vi "GraphMonitor.vi"(8 "error in (no error)":errorcluster, 11 "Connection ID":T2) -> (0 "error out":errorcluster, 3 "Connection ID Out":T2)   [LabVIEW 2017, in "GL860_Driver.lvlib"]
uses:
  GL860_Driver.lvlib
  Driver/ConnectionID.ctl
  D:/src/LabVIEW/GL860/JP/LabView VI/64bitdll/GLSampleProgram.dll
  64bitdll/GLSampleProgram.dll
  Sub/Amp_Param.ctl
panel:
  out "M/C":i32[](array[numeric])
  in  "HEAD":T1 {"FirstPos" format="%<%x %.3X>T"; "Stop" format="%<%x %.3X>T"; "Trig" format="%<%x %.3X>T"; "Start" format="%<%x %.3X>T"}
  out "LogiPul":i32
  out "MaxCH":i32
  out "Unit":bool[](array[boolean])
  out "Bin":i32[](array[numeric])
  out "Reference":refnum<k24>
  out "Pos":i32[](array[numeric])
  out "Idx":i32[](array[numeric])
  out "CH_Size":cluster{"Analog":i32, "Logic":i16, "Pulse":i16}
  in  "閉じる":bool
  in  "一時停止":bool
  out "カーソル値":string
  in  "Ch Select":u16(ring)
  out "Graph":dbl[][](graph)
  # "ALL"
  # "GBD"
  # "CSV"
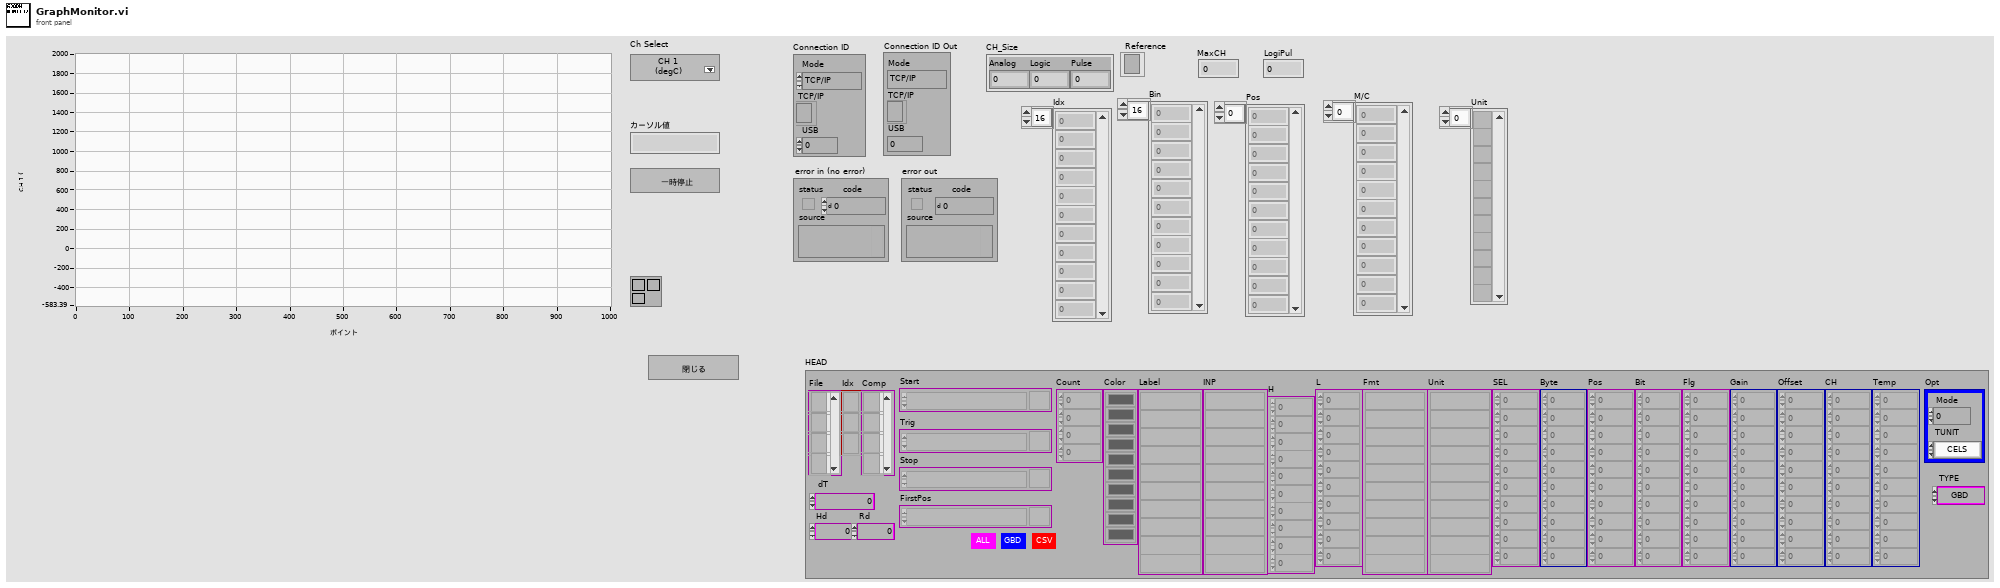
[diagram p1: front panel]
types:
  T1 = typedef "Amp_Param.ctl" = cluster{"File":refnum<file>[], "Idx":refnum<file>[], "dT":dbl, "Hd":i32, "Rd":i32, "Start":timestamp[], "Trig":timestamp[], "Stop":timestamp[], "FirstPos":timestamp[], "Count":i64[], "Color":u32[], "Label":string[], "INP":string[], "H":dbl[], "L":dbl[], "Fmt":string[], "Unit":string[], "SEL":i32[], "Byte":i32[], "Pos":i32[], "Bit":i32[], "Flg":i32[], "Gain":dbl[], "Offset":dbl[], "CH":i32[], "Opt":cluster{"Mode":i32, "TUNIT":enum16{"CELS", "FAHR"}}, "TYPE":enum16{"GBD", "CSV"}, "Comp":refnum<file>[], "Temp":i32[]}
  T2 = typedef "ConnectionID.ctl" = cluster{"Mode":enum16{"TCP/IP", "USB"}, "TCP/IP":refnum<k5>, "USB":i32}
  T3 = cluster{"Meas.Hi":string, "Meas.Lo":string, "Meas.Unit":string, "EU.Hi":string, "EU.Lo":string, "EU.Unit":string}
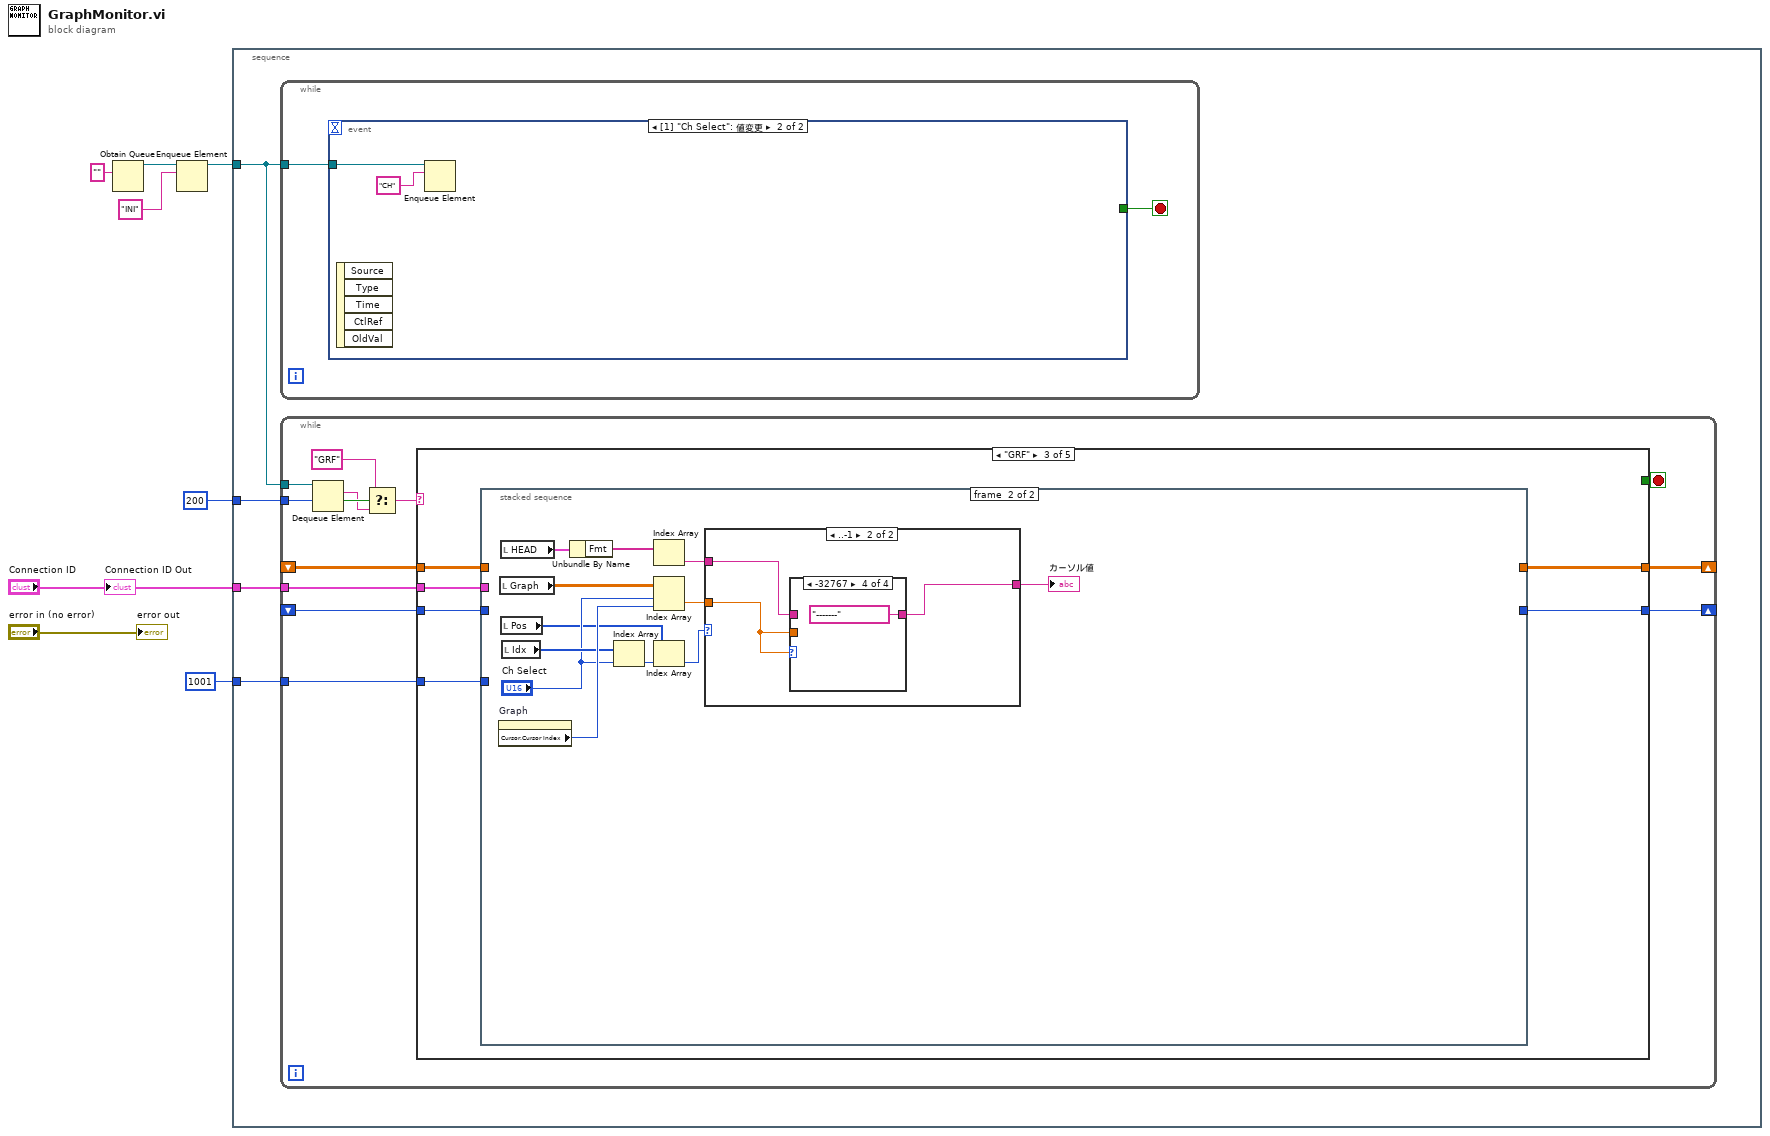
[diagram p0: block diagram]
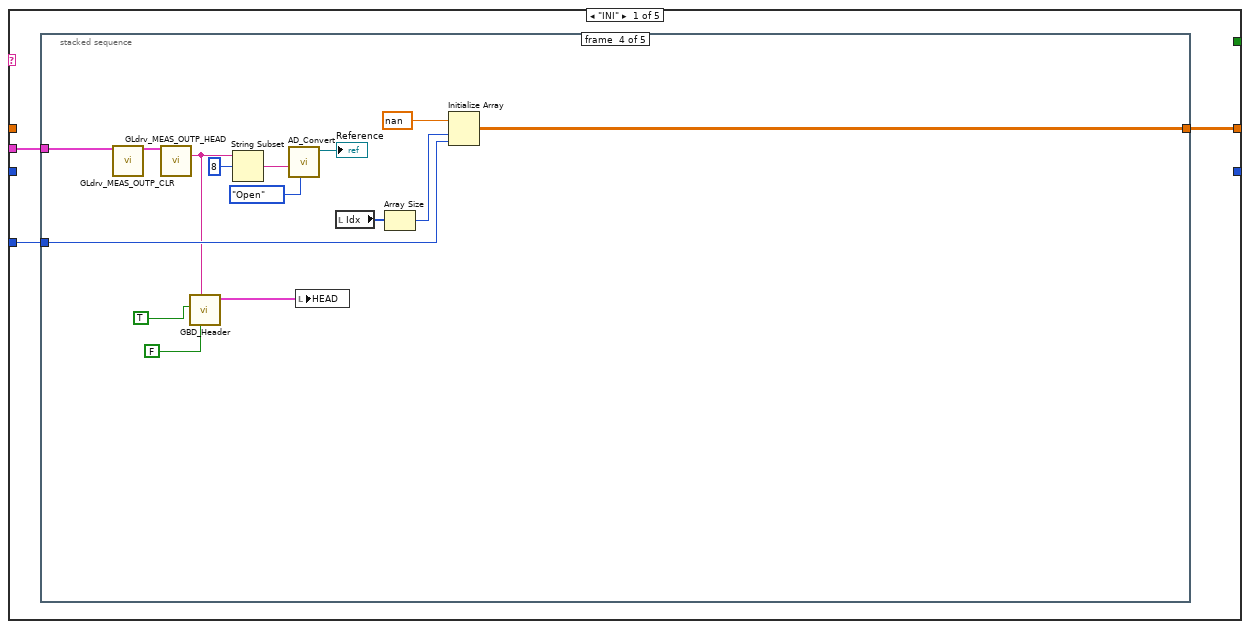
[diagram p2: hidden frame]
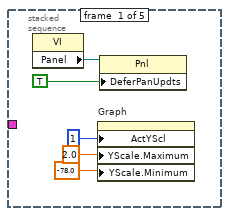
[diagram p3: hidden frame]
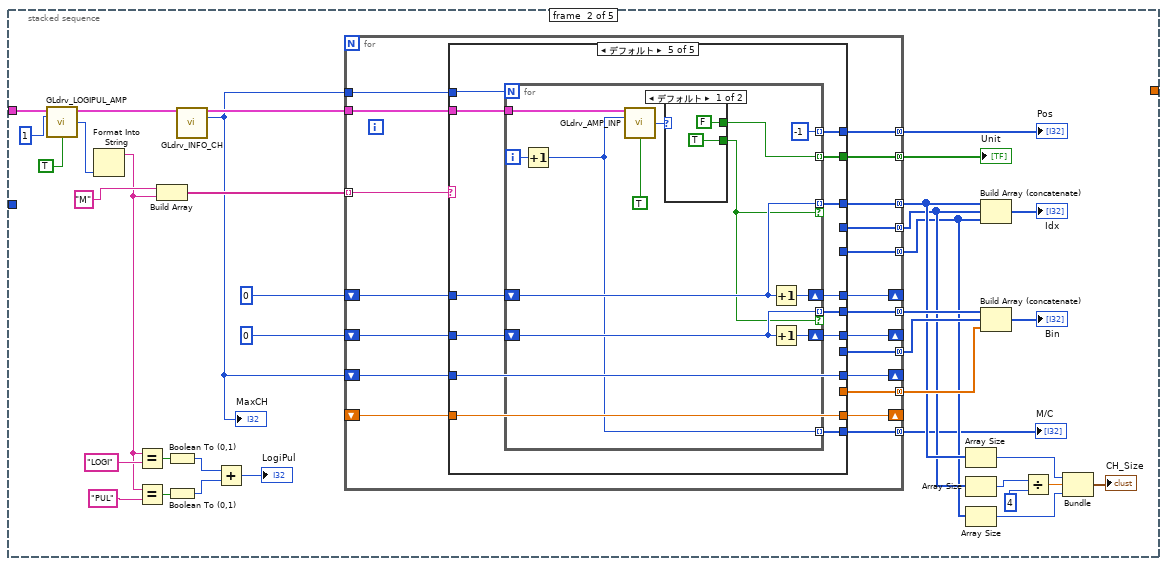
[diagram p4: hidden frame]
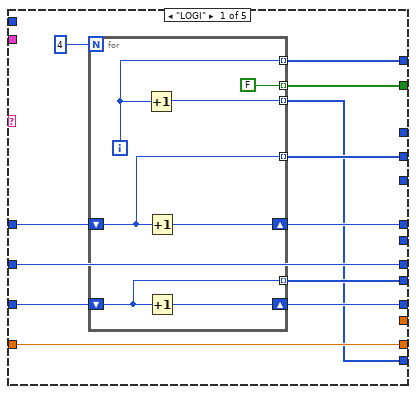
[diagram p5: hidden frame]
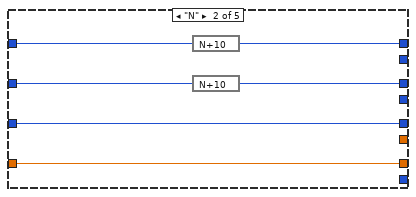
[diagram p6: hidden frame]
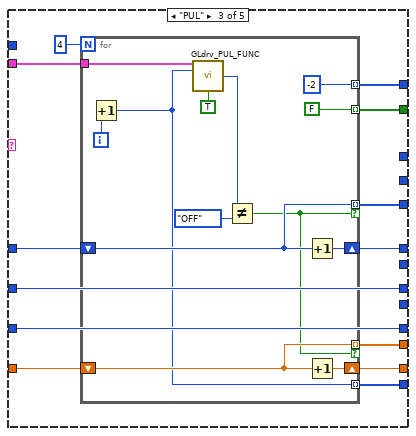
[diagram p7: hidden frame]
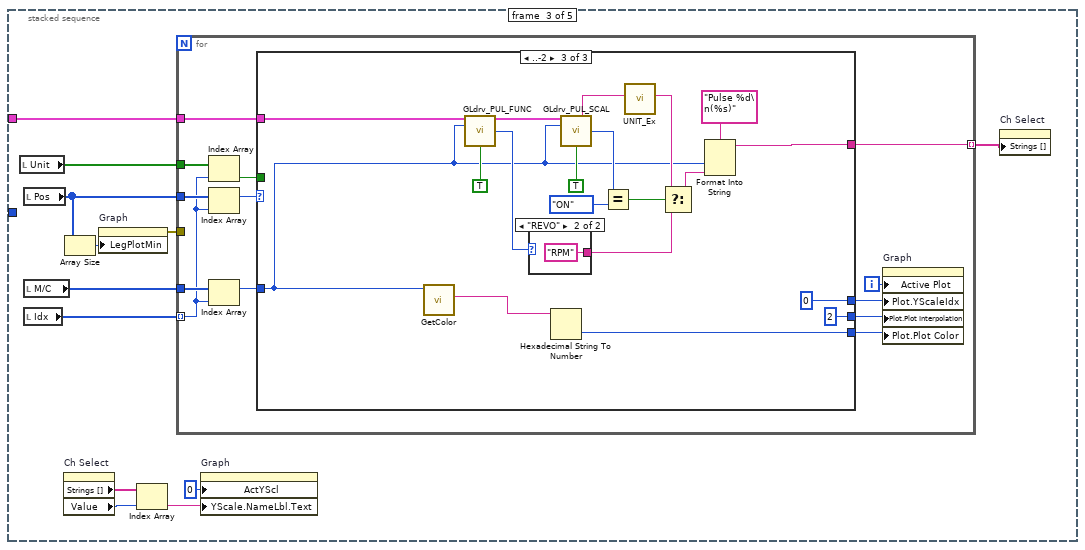
[diagram p10: hidden frame]
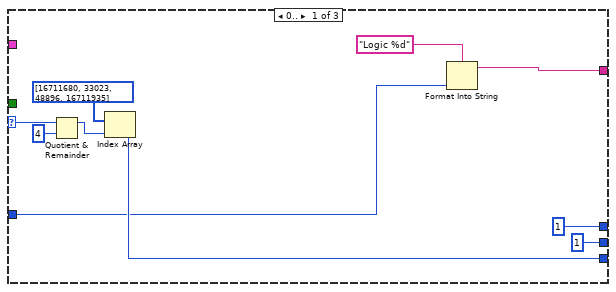
[diagram p11: hidden frame]
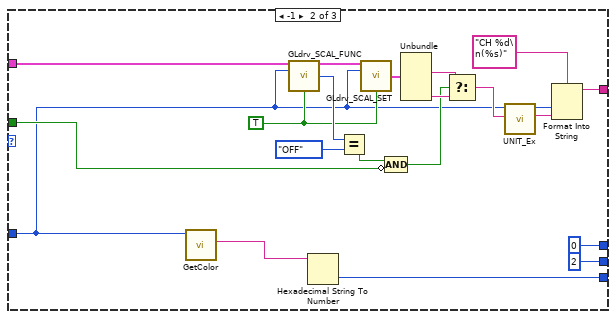
[diagram p12: hidden frame]
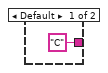
[diagram p13: hidden frame]
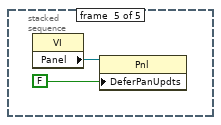
[diagram p14: hidden frame]
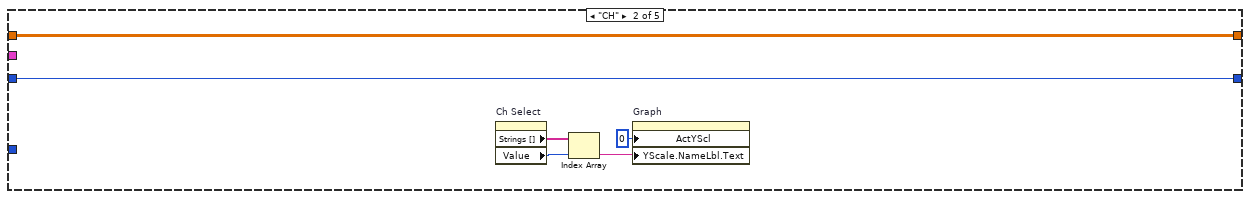
[diagram p15: hidden frame]
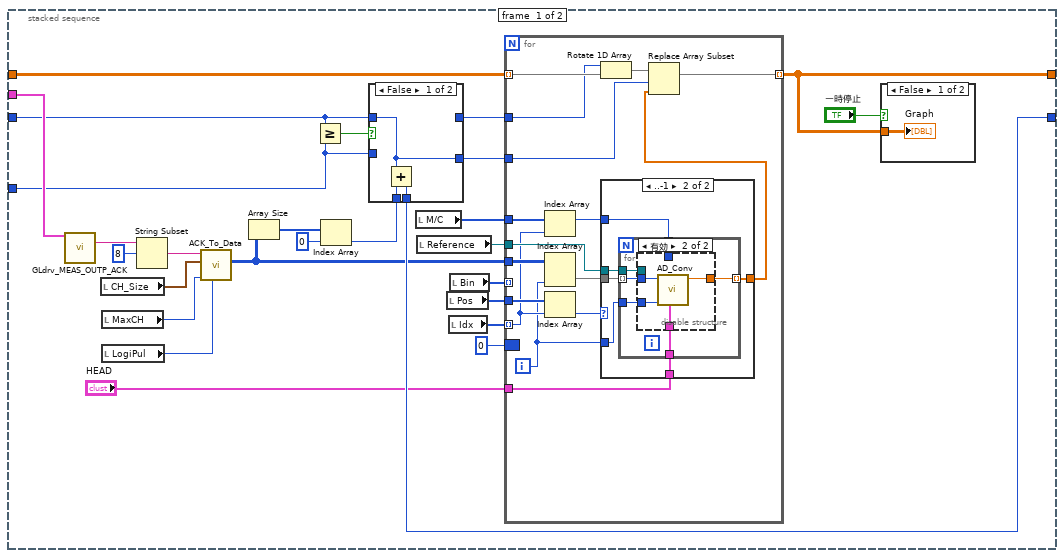
[diagram p16: hidden frame]
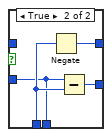
[diagram p18: hidden frame]
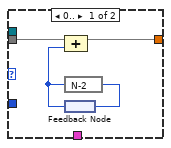
[diagram p19: hidden frame]
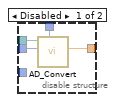
[diagram p20: hidden frame]
diagram:
  n1 = Obtain Queue(element data type="") -> (queue out=w4:refnum<queue>)  [unwired: 4 in, 2 out]
  n2 = Enqueue Element(queue=w4, element="INI") -> (queue out=w3:refnum<queue>)  [unwired: 2 in, 2 out]
  n3 = stacked-sequence {
    tunnel: "Connection ID" -> [w12]
    tunnel: w3 -> [w11]
    tunnel: 200 -> [w10]
    tunnel: 1001 ("dimension size") -> [w9]
    frame #0 {
      n4 = while {
        tunnel: w11 -> [w382]
        stop <- w383 stop-if-true
        n5 = event shown="[1] \"Ch Select\": 値変更" {
          selector: _ -> [_ _]
          dyn-events: _ -> [_ _]
          timeout: _ -> [_ _]
          tunnel: [TRUE _] -> w383
          tunnel: w382 -> [w385 w387]
          event "閉じる": Value Change {
            n6 = event-data() -> ()  [unwired: 1 in, 1 out]
            n7 = Enqueue Element(queue=w385, element="EXIT") -> ()  [unwired: 2 in, 3 out]
          }
          event "Ch Select": Value Change {
            n8 = event-data() -> ()  [unwired: 1 in, 5 out]
            n9 = Enqueue Element(queue=w387, element="CH") -> ()  [unwired: 2 in, 3 out]
          }
        }
      }
      n10 = while {
        tunnel: w11 -> [w25]
        tunnel: w12 -> [w20]
        tunnel: w10 -> [w18]
        shift-right: [w16] -> _
        shift-left: _ -> [w17]
        shift-right: [w15] -> _
        shift-left: _ -> [w14]
        tunnel: w9 -> [w13]
        stop <- w19 stop-if-true
        n11 = Dequeue Element(queue=w25, timeout in ms (-1)=w18) -> (element=w23:string, timed out?=w24:bool)  [unwired: 1 in, 2 out]
        n12 = Select(t="GRF", s=w24, f=w23) -> (s? t:f=w21:string)
        n13 = case shown="\"GRF\"" w21 {
          tunnel: w20 -> [w28 _ w276 _ _]
          tunnel: [_ _ _ TRUE _] -> w19
          tunnel: w17 -> [_ w266 w275 _ _]
          tunnel: [w27 w266 w274 _ _] -> w16
          tunnel: [_ w265 w271 _ _] -> w15
          tunnel: w14 -> [_ w265 w272 _ _]
          tunnel: w13 -> [w26 _ w273 _ _]
          frame "INI" {
            n14 = stacked-sequence {
              tunnel: w28 -> [_ w60 w183 w257 _]
              tunnel: [_ _ _ w255 _] -> w27
              tunnel: w26 -> [_ _ _ w252 _]
              frame #0 {
                n15 = property on="Property Node" class="VI"() -> ("Panel"=w33:refnum<vi>)  [unwired: 2 in, 2 out]
                n16 = property on="Graph" class="WFGraph （指定）"("ActYScl"=1 ("Active Y Scale"), "YScale.Maximum"=2.0 ("Y Scale.Range:Minimum"), "YScale.Minimum"=-78.0 ("Y Scale.Range:Minimum")) -> ()  [unwired: 2 in, 2 out]
                n17 = property on="Property Node" class="Pnl"(reference=w33, "DeferPanUpdts"=TRUE ("Defer Panel Updates")) -> ()  [unwired: 1 in, 2 out]
              }
              frame #1 {
                n18 = call "GLdrv_LOGIPUL_AMP.vi"("Connection ID"=w60, "AMP"=1, "Query(f)"=TRUE) -> ("Connection ID Out"=w55:T2, "Function out"=w58:enum16{"OFF", "LOGI", "PUL"})  [unwired: 10 in, 1 out]
                n19 = Format Into String(w58) -> (resulting string=w45:string)  [unwired: 3 in, 1 out]
                n20 = Equal?(x=w45, y="LOGI") -> (x = y?=w43:bool)
                n21 = Equal?(x=w45, y="PUL") -> (x = y?=w42:bool)
                n22 = Build Array("M", w45) -> (w54:string[])
                n23 = Boolean To (0,1)(Boolean=w43) -> (0, 1=w41:i16)
                n24 = Boolean To (0,1)(Boolean=w42) -> (0, 1=w40:i16)
                n25 = call "GLdrv_INFO_CH.vi"("Connection ID"=w55) -> ("Connection ID Out"=w56:T2, "Analog Size out"=w47:i32)  [unwired: 1 in, 12 out]
                "MaxCH" <- w47
                n26 = Add(x=w41, y=w40) -> (x+y=→"LogiPul":i16)
                n27 = for {
                  tunnel: w56 -> [w89]
                  tunnel: [w70] -> w34 mode=concatenating
                  shift-right: [w87] -> _
                  shift-left: 0 -> [w88]
                  tunnel: [w86] -> w50 mode=concatenating
                  tunnel: [w85] -> w68 mode=concatenating
                  tunnel: [w84] -> w49 mode=concatenating
                  tunnel: [w83] -> w48 mode=concatenating
                  shift-right: [w82] -> _
                  shift-left: 0 -> [w81]
                  shift-right: [w79] -> _
                  shift-left: w47 -> [w80]
                  shift-right: [w78] -> _
                  shift-left: _ -> [w77]
                  tunnel: [w76] -> w65 mode=concatenating
                  tunnel: [w75] -> w64 mode=concatenating
                  tunnel: [w74] -> w63 mode=concatenating
                  tunnel: [w73] -> w61 mode=concatenating
                  tunnel: w54 -> [w72] mode=indexing
                  tunnel: w47 -> [w71]
                  n28 = case shown="デフォルト" w72 {
                    tunnel: w89 -> [_ _ w127 _ w157]
                    tunnel: w88 -> [w98 w114 w123 w144 w154]
                    tunnel: [w99 w113 w122 w144 w155] -> w87
                    tunnel: [_ _ _ _ w156] -> w86
                    tunnel: [w100 _ w125 _ w153] -> w85
                    tunnel: [w97 _ _ _ _] -> w84
                    tunnel: [_ _ w124 _ _] -> w83
                    tunnel: w81 -> [w93 w112 w118 w143 w152]
                    tunnel: [w93 w111 w118 w143 w151] -> w82
                    tunnel: w80 -> [w96 w110 w117 w141 w149]
                    tunnel: [w95 w110 w117 w141 w149] -> w79
                    tunnel: w77 -> [w92 w109 w121 w142 w148]
                    tunnel: [w92 w109 w120 w142 w148] -> w78
                    tunnel: [_ _ _ _ w150] -> w76
                    tunnel: [w94 _ _ _ _] -> w75
                    tunnel: [_ _ w119 _ _] -> w74
                    tunnel: [w91 _ w116 _ w147] -> w73
                    tunnel: w71 -> [_ _ _ _ w146]
                    tunnel: [w90 _ w115 _ w145] -> w70
                    frame "LOGI" {
                      n29 = for {
                        N: 4 -> [_]
                        tunnel: [w102] -> w90 mode=indexing
                        tunnel: [w108] -> w97 mode=indexing
                        shift-right: [w107] -> w99
                        shift-left: w98 -> [w108]
                        tunnel: [w106] -> w100 mode=indexing
                        shift-right: [w105] -> w95
                        shift-left: w96 -> [w104]
                        tunnel: [w104] -> w94 mode=indexing
                        tunnel: [FALSE] -> w91 mode=indexing
                        i -> [w106]
                        n30 = Increment(x=w106) -> (x+1=w102:i32)
                        n31 = Increment(x=w108) -> (x+1=w107:i32)
                        n32 = Increment(x=w104) -> (x+1=w105:i32)
                      }
                    }
                    frame "N" {
                      n33 = expression code="N+10"(w114) -> (w113:i32)
                      n34 = expression code="N+10"(w112) -> (w111:i32)
                    }
                    frame "PUL" {
                      n35 = for {
                        N: 4 -> [_]
                        tunnel: w127 -> [w137]
                        tunnel: [w138] -> w124 mode=indexing if=w130
                        shift-right: [w139] -> w122
                        shift-left: w123 -> [w138]
                        tunnel: [w128] -> w115 mode=indexing
                        tunnel: [-2] -> w125 mode=indexing
                        shift-right: [w132] -> w120
                        shift-left: w121 -> [w131]
                        tunnel: [w131] -> w119 mode=indexing if=w130
                        tunnel: [FALSE] -> w116 mode=indexing
                        i -> [w140]
                        n36 = Increment(x=w140) -> (x+1=w128:i32)
                        n37 = call "GLdrv_PUL_FUNC.vi"("Connection ID"=w137, "CH"=w128, "Query(f)"=TRUE) -> ("Function out"=w136:enum16{"OFF", "COUNT", "REVO", "INST"})  [unwired: 10 in, 2 out]
                        n38 = Not Equal?(x=w136, y=enum16{"OFF", "COUNT", "REVO", "INST"}."OFF") -> (x != y?=w130:bool)
                        n39 = Increment(x=w138) -> (x+1=w139:i32)
                        n40 = Increment(x=w131) -> (x+1=w132:dbl)
                      }
                    }
                    frame "OFF" {
                    }
                    frame Default {
                      n41 = for {
                        N: w146 -> [_]
                        tunnel: w157 -> [w162]
                        shift-right: [w168] -> w155
                        shift-left: w154 -> [w166]
                        tunnel: [w158] -> w145 mode=indexing
                        tunnel: [w166] -> w156 mode=indexing if=w160
                        tunnel: [-1] -> w153 mode=indexing
                        shift-right: [w165] -> w151
                        shift-left: w152 -> [w164]
                        tunnel: [w164] -> w150 mode=indexing if=w160
                        tunnel: [w159] -> w147 mode=indexing
                        i -> [w169]
                        n42 = Increment(x=w169) -> (x+1=w158:i32)
                        n43 = call "GLdrv_AMP_INP.vi"("Connection ID"=w162, "CH"=w158, "Query(f)"=TRUE) -> ("Input out"=w163:enum16{"NONE", "OFF", "DC", "TEMP", "RH"})  [unwired: 2 in, 10 out]
                        n44 = case shown="デフォルト" w163 {
                          tunnel: [TRUE _] -> w160
                          tunnel: [FALSE _] -> w159
                          frame Default {
                          }
                          frame "NONE", "OFF" {
                          }
                        }
                        n45 = Increment(x=w166) -> (x+1=w168:i32)
                        n46 = Increment(x=w164) -> (x+1=w165:i32)
                      }
                    }
                  }
                }
                "Pos" <- w68
                "Unit" <- w61
                "M/C" <- w34
                n47 = Array Size(array=w50) -> (size(s)=w52:i32)
                n48 = Array Size(array=w49) -> (size(s)=w37:i32)
                n49 = Array Size(array=w48) -> (size(s)=w51:i32)
                n50 = Build Array (concatenate)(w50, w49, w48) -> (→"Idx":i32[])
                n51 = Build Array (concatenate)(w65, w64, w63) -> (→"Bin":i32[])
                n52 = Divide(x=w37, y=4) -> (x/y=w36:dbl)
                n53 = Bundle(w52, w36, w51) -> (→"CH_Size":cluster{i32, dbl, i32})  [unwired: 1 out]
              }
              frame #2 {
                n54 = local read "Unit"() -> (w174:bool[])
                n55 = local read "Pos"() -> (w182:i32[])
                n56 = local read "M/C"() -> (w172:i32[])
                n57 = local read "Idx"() -> (w173:i32[])
                n58 = property on="Ch Select" class="Ring （指定）"() -> ("Strings []"=w179:string[], "Value"=w178:u16)  [unwired: 2 in, 2 out]
                n59 = Array Size(array=w182) -> (size(s)=w181:i32)
                n60 = property on="Graph" class="WFGraph （指定）"("LegPlotMin"=w181) -> (error out=w180:errorcluster)  [unwired: 2 in, 1 out]
                n61 = Index Array(array=w179, index=w178) -> (element=w176:string)
                n62 = for {
                  tunnel: w182 -> [w188]
                  tunnel: w183 -> [w196]
                  tunnel: w180 -> [_]
                  tunnel: w172 -> [w190]
                  tunnel: [w191] -> w175 mode=indexing
                  tunnel: w173 -> [w186] mode=indexing
                  tunnel: w174 -> [w185]
                  i -> [w194]
                  n63 = Index Array(array=w185, index=w186) -> (element=w184:bool)
                  n64 = Index Array(array=w188, index=w186) -> (element=w187:i32)
                  n65 = Index Array(array=w190, index=w186) -> (element=w189:i32)
                  n66 = case shown="..-2" w187 {
                    selector: w187 -> [w204 _ _]
                    tunnel: w196 -> [_ w209 w230]
                    tunnel: [w203 w208 w228] -> w195
                    tunnel: [1 2 2] -> w193
                    tunnel: [1 0 0] -> w192
                    tunnel: w189 -> [w197 w207 w227]
                    tunnel: [w199 w217 w242] -> w191
                    tunnel: w184 -> [_ w212 _]
                    frame 0.. {
                      n67 = Quotient & Remainder(x=w204, y=4) -> (x-y*floor(x/y)=w198:i32)  [unwired: 1 out]
                      n68 = Index Array(array=u32[] [16711680, 33023, 48896, 16711935], index=w198) -> (element=w203:u32)
                      n69 = Format Into String(format string="Logic %d", w197) -> (resulting string=w199:string)  [unwired: 2 in, 1 out]
                    }
                    frame -1 {
                      w221 = TRUE ("Query(f)")
                      n70 = call "GetColor.vi"("CH"=w207) -> ("Strings"=w210:string)  [unwired: 9 in]
                      n71 = call "GLdrv_SCAL_FUNC.vi"("Connection ID"=w209, "CH"=w207, "Query(f)"=w221) -> ("Connection ID Out"=w224:T2, "Function out"=w223:enum16{"ON", "OFF"})  [unwired: 10 in, 1 out]
                      n72 = Hexadecimal String To Number(string=w210) -> (number=w208:u32)  [unwired: 2 in, 1 out]
                      n73 = Equal?(x=w223, y=enum16{"ON", "OFF"}."OFF") -> (x = y?=w213:bool)
                      n74 = call "GLdrv_SCAL_SET.vi"("Connection ID"=w224, "CH"=w207, "Query(f)"=w221) -> ("Scale out"=w220:T3)  [unwired: 10 in, 2 out]
                      n75 = Compound Arithmetic op=AND(w213, invert w212) -> (w214:bool)
                      n76 = Unbundle(w220) -> ("Meas.Unit"=w215:string, "EU.Unit"=w219:string)  [unwired: 4 out]
                      n77 = Select(t=w215, s=w214, f=w219) -> (s? t:f=w216:string)
                      n78 = call "UNIT_Ex.vi"("In"=w216) -> ("Out"=w211:string)  [unwired: 10 in]
                      n79 = Format Into String(format string="CH %d\n(%s)", w207, w211) -> (resulting string=w217:string)  [unwired: 2 in, 1 out]
                    }
                    frame ..-2 {
                      n80 = call "GetColor.vi"("CH"=w227) -> ("Strings"=w229:string)  [unwired: 9 in]
                      n81 = call "GLdrv_PUL_FUNC.vi"("Connection ID"=w230, "CH"=w227, "Query(f)"=TRUE) -> ("Connection ID Out"=w240:T2, "Function out"=w238:enum16{"OFF", "COUNT", "REVO", "INST"})  [unwired: 10 in, 1 out]
                      n82 = case shown="\"REVO\"" w238 {
                        tunnel: ["C" ("data out") "RPM" ("data out")] -> w234
                        frame Default {
                        }
                        frame "REVO" {
                        }
                      }
                      n83 = Hexadecimal String To Number(string=w229) -> (number=w228:u32)  [unwired: 2 in, 1 out]
                      n84 = call "GLdrv_PUL_SCAL.vi"("Connection ID"=w240, "CH"=w227, "Query(f)"=TRUE) -> ("Unit out"=w232:string, "Function out"=w237:enum16{"ON", "OFF"})  [unwired: 7 in, 4 out]
                      n85 = Equal?(x=w237, y=enum16{"ON", "OFF"}."ON") -> (x = y?=w235:bool)
                      n86 = call "UNIT_Ex.vi"("In"=w232) -> ("Out"=w231:string)  [unwired: 10 in]
                      n87 = Select(t=w231, s=w235, f=w234) -> (s? t:f=w233:string)
                      n88 = Format Into String(format string="Pulse %d\n(%s)", w227, w233) -> (resulting string=w242:string)  [unwired: 2 in, 1 out]
                    }
                  }
                  n89 = property on="Graph" class="WFGraph （指定）"("Active Plot"=w194, "Plot.YScaleIdx"=w192, "Plot.Plot Interpolation"=w193, "Plot.Plot Color"=w195) -> ()  [unwired: 2 in, 2 out]
                }
                n90 = property on="Graph" class="WFGraph （指定）"("ActYScl"=0 ("Active Y Scale"), "YScale.NameLbl.Text"=w176) -> ()  [unwired: 2 in, 2 out]
                n91 = property on="Ch Select" class="Ring （指定）"("Strings []"=w175) -> ()  [unwired: 2 in, 2 out]
              }
              frame #3 {
                n92 = call "GLdrv_MEAS_OUTP_CLR.vi"("Connection ID"=w257) -> ("Connection ID Out"=w258:T2)  [unwired: 12 in, 2 out]
                n93 = call "GLdrv_MEAS_OUTP_HEAD.vi"("Connection ID"=w258) -> ("Header out"=w250:string)  [unwired: 12 in, 2 out]
                n94 = call "GBD_Header.vi"("Head"=w250, "Save?"=FALSE, "Cvt_Mode"=TRUE) -> ("Param"=w249:T1)  [unwired: 4 in, 4 out]
                n95 = String Subset(string=w250, offset (0)=8) -> (substring=w259:string)  [unwired: 1 in]
                n96 = call "AD_Convert.vi"("Mode"=enum16{"Open", "Convert", "Close"}."Open", "Header"=w259) -> ("Reference.Out"=→"Reference":refnum<k24>)  [unwired: 7 in, 2 out]
                n97 = local write "HEAD"(w249) -> ()
                n98 = local read "Idx"() -> (w254:i32[])
                n99 = Array Size(array=w254) -> (size(s)=w253:i32)
                n100 = Initialize Array(nan, w253, w252) -> (w255:dbl[][])
              }
              frame #4 {
                n101 = property on="Property Node" class="VI"() -> ("Panel"=w264:refnum<vi>)  [unwired: 2 in, 2 out]
                n102 = property on="Property Node" class="Pnl"(reference=w264, "DeferPanUpdts"=FALSE ("Defer Panel Updates")) -> ()  [unwired: 1 in, 2 out]
              }
            }
          }
          frame "CH" {
            n103 = property on="Ch Select" class="Ring （指定）"() -> ("Strings []"=w270:string[], "Value"=w269:u16)  [unwired: 2 in, 2 out]
            n104 = Index Array(array=w270, index=w269) -> (element=w267:string)
            n105 = property on="Graph" class="WFGraph （指定）"("ActYScl"=0 ("Active Y Scale"), "YScale.NameLbl.Text"=w267) -> ()  [unwired: 2 in, 2 out]
          }
          frame "GRF" {
            n106 = stacked-sequence {
              tunnel: w276 -> [w303 _]
              tunnel: w275 -> [w300 _]
              tunnel: [w285 _] -> w274
              tunnel: w273 -> [w296 _]
              tunnel: w272 -> [w294 _]
              tunnel: [w291 _] -> w271
              frame #0 {
                n107 = call "GLdrv_MEAS_OUTP_ACK.vi"("Connection ID"=w303) -> ("Data out"=w302:string)  [unwired: 12 in, 2 out]
                n108 = local read "CH_Size"() -> (w301:cluster{"Analog":i32, "Logic":i16, "Pulse":i16})
                n109 = local read "MaxCH"() -> (w281:i32)
                n110 = local read "LogiPul"() -> (w280:i32)
                n111 = String Subset(string=w302, offset (0)=8) -> (substring=w279:string)  [unwired: 1 in]
                n112 = call "ACK_To_Data.vi"("LogiPul"=w280, "MaxCH"=w281, "Size"=w301, "String"=w279) -> ("Bin_Data_All"=w287:i32[][])  [unwired: 6 in, 1 out]
                n113 = Array Size(array=w287) -> (size(s)=w299:i32[])
                n114 = Greater Or Equal?(x=w294, y=w296) -> (x >= y?=w295:bool)
                n115 = Index Array(array=w299, index=0) -> (element=w297:i32)
                n116 = case shown="FALSE" w295 {
                  tunnel: w296 -> [_ w308]
                  tunnel: w297 -> [w306 w311]
                  tunnel: w294 -> [w307 _]
                  tunnel: [_ w310] -> w293
                  tunnel: [w307 w309] -> w292
                  tunnel: [w305 w308] -> w291
                  frame False {
                    n117 = Add(x=w307, y=w306) -> (x+y=w305:i32)
                  }
                  frame True {
                    n118 = Negate(x=w311) -> (-x=w310:i32)
                    n119 = Subtract(x=w308, y=w311) -> (x-y=w309:i32)
                  }
                }
                n120 = local read "M/C"() -> (w277:i32[])
                n121 = local read "Reference"() -> (w284:refnum<k24>)
                n122 = local read "Pos"() -> (w288:i32[])
                n123 = local read "Idx"() -> (w289:i32[])
                n124 = local read "Bin"() -> (w283:i32[])
                n125 = for {
                  tunnel: w287 -> [w326]
                  tunnel: w300 -> [w327] mode=indexing
                  tunnel: [w325] -> w285 mode=indexing
                  tunnel: w293 -> [w323]
                  tunnel: w292 -> [w322]
                  tunnel: w289 -> [w313] mode=indexing
                  tunnel: w288 -> [w317]
                  tunnel: w277 -> [w319]
                  tunnel: w284 -> [w320]
                  tunnel: w283 -> [_] mode=indexing
                  border: 0 -> [_]
                  tunnel: "HEAD" -> [w314]
                  i -> [w312]
                  n126 = Index Array(array=w319, index=w313) -> (element=w318:i32)
                  n127 = Index Array(array=w326, index (col)=w312) -> (element=w324:i32[])  [unwired: 1 in]
                  n128 = Index Array(array=w317, index=w313) -> (element=w316:i32)
                  n129 = Rotate 1D Array(1:w327, 2:w323) -> (0:w321:dbl[])
                  n130 = case shown="..-1" w316 {
                    tunnel: w324 -> [w331 w337]
                    tunnel: [w330 w336] -> w315
                    tunnel: w320 -> [_ w335]
                    tunnel: w318 -> [_ w332]
                    tunnel: w314 -> [_ w334]
                    tunnel: w312 -> [_ w333]
                    frame 0.. {
                      n131 = feedback #1() -> (w329:i32)
                      n132 = Compound Arithmetic op=ADD(w331, w329) -> (w330:i32[])
                      n133 = expression code="N-2"(w329) -> (w328:i32)
                      n134 = feedback-in #1(w328) -> ()
                    }
                    frame ..-1 {
                      n135 = for {
                        tunnel: w337 -> [w341] mode=indexing
                        tunnel: [w340] -> w336 mode=indexing
                        tunnel: w332 -> [w343]
                        tunnel: w335 -> [w342]
                        tunnel: w334 -> [w339]
                        tunnel: w333 -> [w338]
                        n136 = disable-structure shown="有効" {
                          disable-tunnel: w343 -> [w347 _]
                          disable-tunnel: w342 -> [w346 _]
                          disable-tunnel: w341 -> [w345 w351]
                          disable-tunnel: [w344 w350] -> w340
                          disable-tunnel: w339 -> [_ w349]
                          disable-tunnel: w338 -> [_ w348]
                          frame Disabled {
                            n137 = call "AD_Convert.vi"("CH"=w347, "Data"=w345, "Reference.In"=w346) -> ("AD"=w344:dbl)  [unwired: 6 in, 2 out]
                          }
                          frame Enabled {
                            n138 = call "AD_Conv.vi"("HEAD"=w349, "No"=w348, "ACK"=w351) -> ("Data"=w350:dbl)  [unwired: 8 in]
                          }
                        }
                      }
                    }
                  }
                  n139 = Replace Array Subset(array=w321, new element=w315, index=w322) -> (w325:dbl[])
                }
                n140 = case shown="FALSE" "一時停止" {
                  tunnel: w285 -> [w304 _]
                  frame False {
                    "Graph" <- w304
                  }
                  frame True {
                  }
                }
              }
              frame #1 {
                n141 = property on="Graph" class="WFGraph （指定）"() -> ("Cursor.Cursor Index"=w363:i32)  [unwired: 2 in, 2 out]
                n142 = local read "Graph"() -> (w359:dbl[][])
                n143 = local read "HEAD"() -> (w354:T1)
                n144 = local read "Pos"() -> (w356:i32[])
                n145 = local read "Idx"() -> (w360:i32[])
                n146 = Unbundle By Name(w354) -> ("Fmt"=w353:string[])
                n147 = Index Array(array=w360, index="Ch Select") -> (element=w357:i32)
                n148 = Index Array(array=w353) -> (element=w352:string)  [unwired: 1 in]
                n149 = Index Array(array=w359, index (row)="Ch Select", index (col)=w363) -> (element=w361:dbl)
                n150 = Index Array(array=w356, index=w357) -> (element=w355:i32)
                n151 = case shown="..-1" w355 {
                  tunnel: w361 -> [w369 w370]
                  tunnel: [w365 w372] -> w362
                  tunnel: w352 -> [_ w371]
                  frame 0.. {
                    n152 = To Long Integer(number=w369) -> (32bit integer=w368:i32)
                    n153 = And(x=w368, y=1) -> (x .and. y?=w366:i32)
                    n154 = Index Array(array=string[] ["L", "H"], index=w366) -> (element=w365:string)
                  }
                  frame ..-1 {
                    n155 = case shown="-32767" w370 {
                      tunnel: w370 -> [w375 _ _ _]
                      tunnel: [w374 "BURNOUT" "+++++++" "-------"] -> w372
                      tunnel: w371 -> [w373 _ _ _]
                      frame Default {
                        n156 = Format Into String(format string=w373, w375) -> (resulting string=w374:string)  [unwired: 2 in, 1 out]
                      }
                      frame 32765 {
                      }
                      frame 32764 {
                      }
                      frame -32767 {
                      }
                    }
                  }
                }
                "カーソル値" <- w362
              }
            }
          }
          frame "EXIT" {
            n157 = local read "Reference"() -> (w379:refnum<k24>)
            n158 = call "AD_Convert.vi"("Mode"=enum16{"Open", "Convert", "Close"}."Close", "Reference.In"=w379) -> ()  [unwired: 7 in, 3 out]
          }
          frame Default {
          }
        }
      }
    }
  }
  "error out" <- "error in (no error)"
  "Connection ID Out" <- "Connection ID"
